vi "Histogram Plot.vi"() -> ()   [LabVIEW 2023]
doc: "Uses a bar plot type of waveform graph to draw a histogram of randomly generated data by calling the Plot Waveform VI. Each iteration of the loop adds new data to the histogram."
uses:
  <vilib>/picture/cartesn2.llb/Waveform Plot Type.ctl
panel:
  out "Generated Data":dbl(graph)
  in  "Stop":bool
  out "Histogram":picture
  # "Overview: Uses the Plot Waveform VI with a 'bar plot' waveform type to draw a histogram of random data.\nInstructions:\n1. Run the VI.\n2. Click Stop to stop the VI."
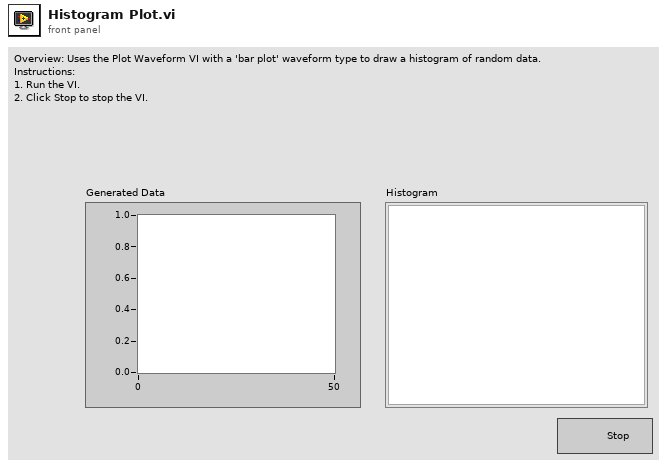
[diagram p1: front panel]
types:
  T1 = cluster{"line color":u32, "text color":u32, "tick length(3)":i16, "crossing axes":bool, "visible grid?":bool}
  T2 = cluster{"x minimum":dbl, "x maximum":dbl, "x log?":bool, "x precision":u8, "x format":enum8{"Decimal", "Scientific", "Engineering", "Binary", "Octal", "Hex"}, "y minimum":dbl, "y maximum":dbl, "y log?":bool, "y precision":u8, "y format":enum8{"Decimal", "Scientific", "Engineering", "Binary", "Octal", "Hex"}}
  T3 = typedef "Waveform Plot Type.ctl" = enum16{"points", "squares", "circles", "connected points", "connected squares", "connected circles", "fill to baseline", "comb plot", "bar plot"}
  T4 = cluster{"plot color":u32, "plot type":T3, "baseline":dbl}
  T5 = typedef "LVBoundsTypeDef.ctl" = cluster{"Width":u32, "Height":u32}
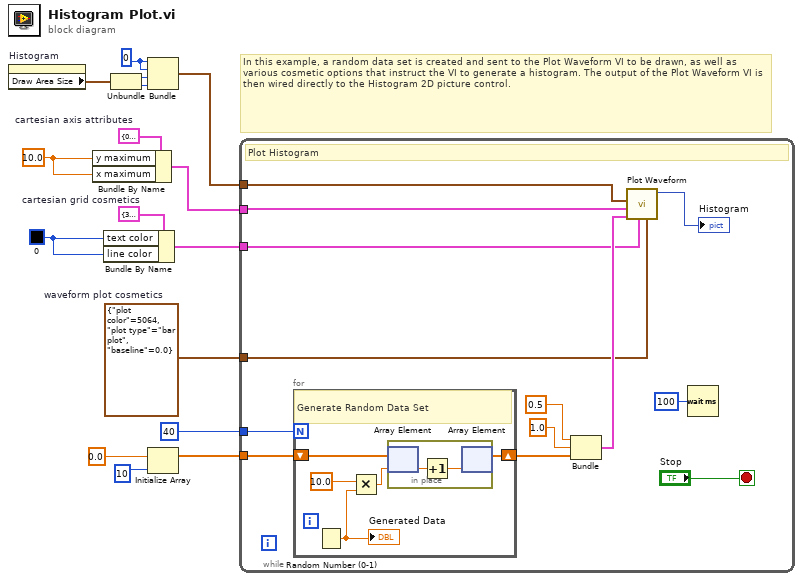
[diagram p0: block diagram]
diagram:
  w3 = u32 0
  w5 = T1 {"line color"=39168, "text color"=65280, "tick length(3)"=3, "crossing axes"=FALSE, "visible grid?"=TRUE}  # cartesian grid cosmetics
  w6 = T2 {"x minimum"=0.0, "x maximum"=0.0, "x log?"=FALSE, "x precision"=1, "x format"=enum."Decimal", "y minimum"=0.0, "y maximum"=0.0, "y log?"=FALSE, "y precision"=1, "y format"=enum."Decimal"}  # cartesian axis attributes
  w7 = 10.0 ("x maximum")
  w8 = T4 {"plot color"=5064, "plot type"=enum."bar plot", "baseline"=0.0}  # waveform plot cosmetics
  w11 = 0
  # "In this example, a random data set is created and sent to the Plot Waveform VI to be drawn, as well as various cosmetic options that instruct the VI to generate a histogram. The output of the Plot Waveform VI is then wired directly to the Histogram 2D picture control."
  n1 = property on="Histogram" class="Pict"() -> ("Draw Area Size"=w14:T5)  [unwired: 2 in, 2 out]
  n2 = Bundle By Name(cluster=w6, "y maximum"=w7, "x maximum"=w7) -> (w2:T2)
  n3 = Bundle By Name(cluster=w5, "text color"=w3, "line color"=w3) -> (w4:T1)
  n4 = Unbundle(w14) -> ("Width"=w12:u32, "Height"=w13:u32)
  n5 = Bundle(w11, w11, "Width"=w12, "Height"=w13) -> (w10:cluster{i32, i32, "Width":u32, "Height":u32})  [unwired: 1 in]
  n6 = Initialize Array(0.0, 10) -> (w15:dbl[])
  n7 = while {
    tunnel: w10 -> [w27]
    tunnel: w15 -> [w28]
    tunnel: 40 ("Points in Each Histogram") -> [w23]
    tunnel: w2 -> [w21]
    tunnel: w8 -> [w20]
    tunnel: w4 -> [w19]
    stop <- "Stop" stop-if-true
    # "Plot Histogram"
    n8 = for {
      N: w23 -> [_]
      shift-right: [w32] -> w29
      shift-left: w28 -> [w31]
      # "Generate Random Data Set"
      n9 = Random Number (0-1)() -> (number: 0 to 1=w34:dbl)
      "Generated Data" <- w34
      n10 = Multiply(x=10.0, y=w34) -> (x*y=w33:dbl)
      n11 = in-place {
        n12 = in-place-array #1(w31, w33) -> (w36:dbl)
        n13 = Increment(x=w36) -> (x+1=w35:dbl)
        n14 = in-place-array #1(w35) -> (w32:dbl[])  [unwired: 1 out]
      }
    }
    n15 = Bundle(0.5, 1.0, w29) -> (w26:cluster{dbl, dbl, dbl[]})  [unwired: 1 in]
    n16 = call <vilib>:"Plot Waveform.vi"("waveform plot cosmetics"=w20, "cartesian grid cosmetics"=w19, "waveform data"=w26, "cartesian axis attributes"=w21, "bounding rect"=w27) -> ("new picture"=→"Histogram":picture)  [unwired: 6 in]
    n17 = Wait (ms)(milliseconds to wait=u32 100) -> ()  [unwired: 1 out]
  }
